vi "Snake location.vi"(8 "error in (no error)":errorcluster, 10 "Snake location":T1[](array[typedef]), 11 "Snake in":refnum<class "Snake.lvclass">) -> (0 "error out":errorcluster, 3 "Snake out":refnum<class "Snake.lvclass">)   [LabVIEW 2021, in "Snake.lvclass"]
uses:
  Snake.lvclass
  Position.ctl
  Snake.lvclass/Snake.ctl
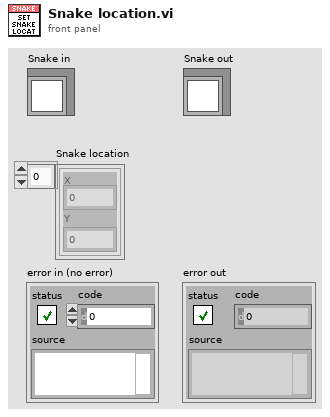
[diagram p1: front panel]
types:
  T1 = typedef "Position.ctl" = cluster{"X":u32, "Y":u32}
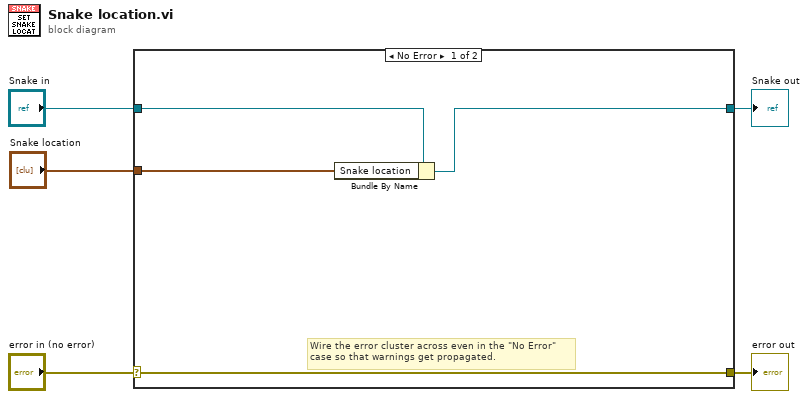
[diagram p0: block diagram]
diagram:
  n1 = case shown="No Error" "error in (no error)" {
    selector: "error in (no error)" -> [w8 w11]
    tunnel: [w8 w11] -> w4
    tunnel: [w7 w10] -> w2
    tunnel: "Snake in" -> [w9 w10]
    tunnel: "Snake location" -> [w6 _]
    frame No Error {
      # "Wire the error cluster across even in the \"No Error\"\ncase so that warnings get propagated."
      n2 = Bundle By Name(cluster=w9, "Snake location"=w6) -> (w7:refnum<class "Snake.lvclass">)
    }
    frame Error {
    }
  }
  "error out" <- w4
  "Snake out" <- w2
